vi "App.Initialize.vi"(8 "error in (no error)":errorcluster, 11 "Start Variables":T1={"Aliases.All"=[], "Aliases.Outputs"=[], "UI.Sequence#ofColumns"=0, "SysDef.Path"=path "", "UI.SequenceRef"=refnum, "UI.StepInformationRef"=refnum, "UI.AbortRef"=refnum, "UI.GraphRef"=refnum, "UI.ViewRef"=refnum, "UI.IterationsRef"=refnum, "UI.IterationInformationRef"=refnum, "INI.Settings"={"Build Location"=path "C:/Simple Sequence Editor/SequenceRepo", "LoggingLocation"=path ""}}) -> (0 "error out":errorcluster)   [LabVIEW 2013, in "Simple Sequence Tools - Editor.lvlib"]
uses:
  Simple Sequence Tools - Editor.lvlib
  Types/StateVariables.ctl
  Shared/Types/ChannelProperties.ctl
  Shared/Types/INI.Settings
  Types/UI.PropertiesTypes.ctl
  Shared/SubVIs/Constants.vi
  Shared/Simple Sequence Tools - Shared.lvlib
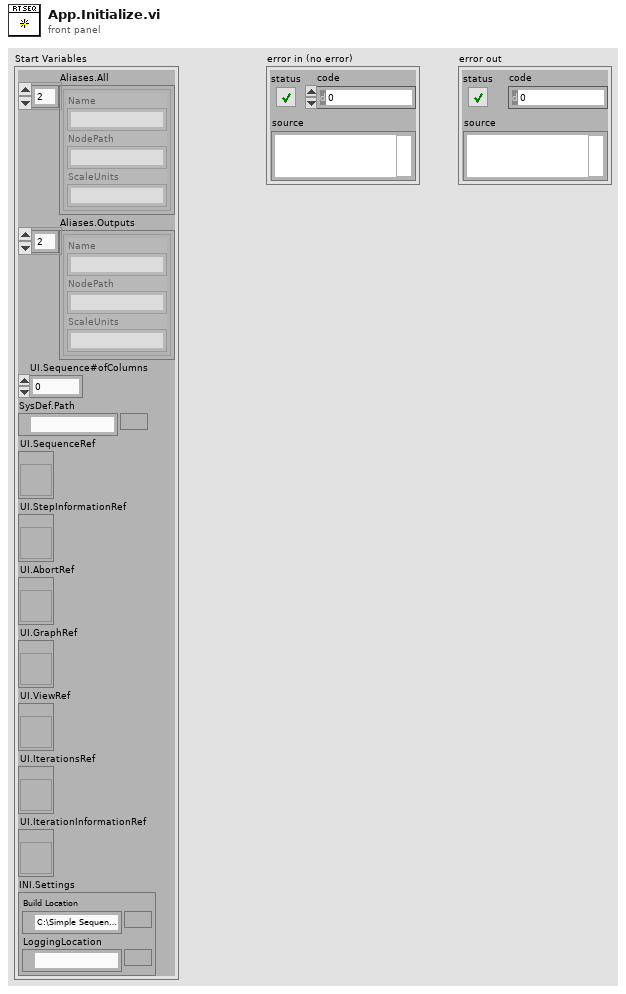
[diagram p1: front panel]
types:
  T1 = typedef "Simple Sequence Tools - Editor.lvlib/StateVariables.ctl" = cluster{"Aliases.All":T2[], "Aliases.Outputs":T2[], "UI.Sequence#ofColumns":i32, "SysDef.Path":path, "UI.SequenceRef":refnum<vi>, "UI.StepInformationRef":refnum<vi>, "UI.AbortRef":refnum<vi>, "UI.GraphRef":refnum<vi>, "UI.ViewRef":refnum<vi>, "UI.IterationsRef":refnum<vi>, "UI.IterationInformationRef":refnum<vi>, "INI.Settings":T3}
  T2 = typedef "Simple Sequence Tools - Shared.lvlib/ChannelProperties.ctl" = cluster{"Name":string, "NodePath":string, "ScaleUnits":string}
  T3 = typedef "Simple Sequence Tools - Shared.lvlib/INI.Settings" = cluster{"Build Location":path, "LoggingLocation":path}
  T4 = typedef "Simple Sequence Tools - Editor.lvlib/UI.PropertiesTypes.ctl" = enum8{"Step Properties", "Sequence Properties"}
  T5 = typedef "LVBoundsTypeDef.ctl" = cluster{"Width":u32, "Height":u32}
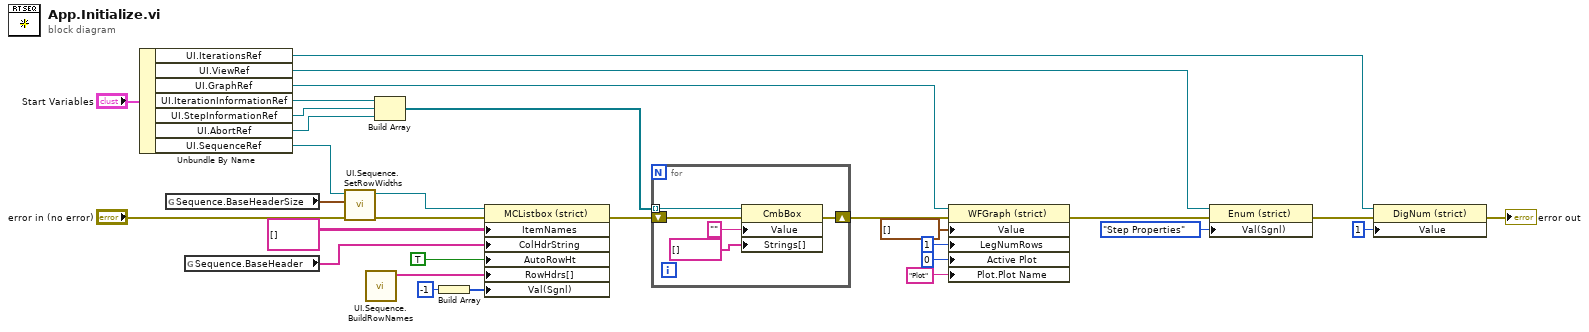
[diagram p0: block diagram]
diagram:
  n1 = Unbundle By Name("Start Variables") -> ("UI.IterationsRef"=w5:refnum<vi>, "UI.ViewRef"=w27:refnum<vi>, "UI.GraphRef"=w21:refnum<vi>, "UI.IterationInformationRef"=w1:refnum<vi>, "UI.StepInformationRef"=w19:refnum<vi>, "UI.AbortRef"=w18:refnum<vi>, "UI.SequenceRef"=w13:refnum<vi>)
  n2 = global read "Constants.vi" "Sequence.BaseHeaderSize"() -> (w6:T5[])
  n3 = global read "Constants.vi" "Sequence.BaseHeader"() -> (w7:string[])
  n4 = call "UI.Sequence.SetRowWidths.vi"("error in (no error)"="error in (no error)", "CellSize"=w6, "UI.SequenceRef"=w13) -> ("error out"=w12:errorcluster, "UI.SequenceRef"=w14:refnum<vi>)  [unwired: 7 in]
  n5 = call "UI.Sequence.BuildRowNames.vi"() -> ("Row Headings"=w15:string[])  [unwired: 11 in]
  n6 = Build Array(w1, w19, w18) -> (w20:refnum<vi>[])
  n7 = Build Array(-1 ("Value")) -> (w17:i32[])
  n8 = property class="MCListbox (strict)"(reference=w14, error in=w12, "ItemNames"=string[][] [] ("Item Names"), "ColHdrString"=w7, "AutoRowHt"=TRUE ("Autosizing Row Height"), "RowHdrs[]"=w15, "Val(Sgnl)"=w17) -> (error out=w30:errorcluster)  [unwired: 1 out]
  n9 = for {
    tunnel: w20 -> [w34] mode=indexing
    shift-right: [w32] -> w22
    shift-left: w30 -> [w35]
    n10 = property class="CmbBox"(reference=w34, error in=w35, "Value"="", "Strings[]"=string[] [] ("Strings []")) -> (error out=w32:errorcluster)  [unwired: 1 out]
  }
  n11 = property class="WFGraph (strict)"(reference=w21, error in=w22, "Value"=waveform(dbl)[] [], "LegNumRows"=u32 1 ("Legend:Number of Rows"), "Active Plot"=u32 0, "Plot.Plot Name"="Plot") -> (error out=w28:errorcluster)  [unwired: 1 out]
  n12 = property class="Enum (strict)"(reference=w27, error in=w28, "Val(Sgnl)"=UI.PropertiesTypes."Step Properties" ("Value (Signaling)")) -> (error out=w4:errorcluster)  [unwired: 1 out]
  n13 = property class="DigNum (strict)"(reference=w5, error in=w4, "Value"=u32 1) -> (error out=→"error out":errorcluster)  [unwired: 1 out]
